vi "170519018sinyal_jenaretörü.vi"() -> ()   [LabVIEW 2020]
uses:
  <vilib>/measure/NI_MABase.lvlib
panel:
  out "DALGA FORMUNUN GRAFIGI":waveform(dbl)(graph)
  in  "kare dalga/square  wave duty cycle (%)":dbl(knob)=50.0 scale=0.0..100.0
  in  "offset":dbl(knob) scale=0.0..10.0
  in  "sinyal tipi-signal type":T1(ring)
  in  "GENLIK":dbl(knob)=1.0 scale=0.0..10.0
  in  "FREKANS":dbl(knob)=10.0 scale=0.0..10.0
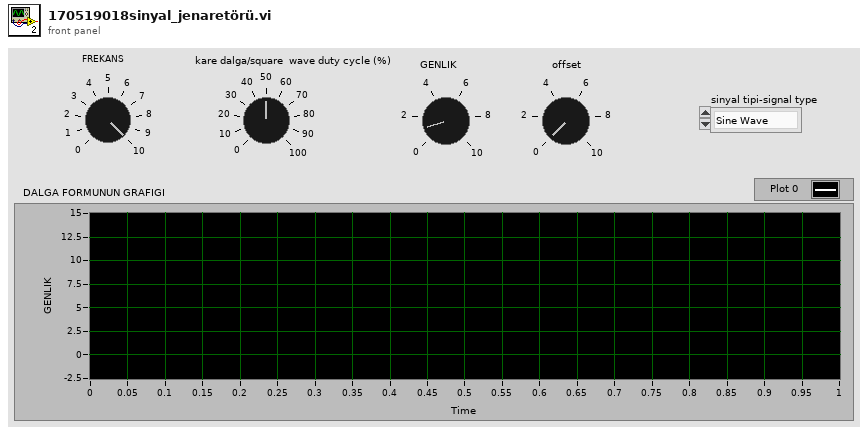
[diagram p1: front panel]
types:
  T1 = enum16{"Sine Wave", "Triangle Wave", "Square Wave", "Sawtooth Wave"}
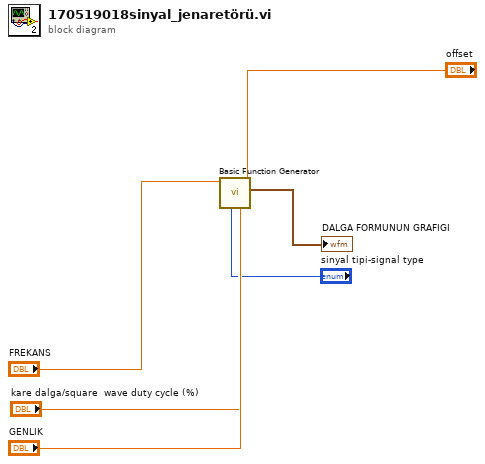
[diagram p0: block diagram]
diagram:
  n1 = call <vilib>:"Basic Function Generator.vi"("offset"="offset", "square wave duty cycle (%)"="kare dalga/square  wave duty cycle (%)", "signal type"="sinyal tipi-signal type", "phase"="sinyal tipi-signal type", "amplitude"="GENLIK", "frequency"="FREKANS") -> ("signal out"=→"DALGA FORMUNUN GRAFIGI":waveform(dbl))  [unwired: 3 in, 2 out]
